vi "channel create.vi"(6 "channel classification (output data)":T1=enum."output data", 9 "data type":T2, 10 "channel name":string) -> (3 "channel":refnum<class "TBM channel.lvclass">)   [LabVIEW 2013, in "file io module configuration.lvclass"]
uses:
  file io module configuration.lvclass
  <vilib>/NI/Tag Bus/tag/Data Type.ctl
  <vilib>/NI/Tag Bus Module Framework/channel/TBM channel.lvclass
  <vilib>/NI/Tag Bus Module Framework/channel/channel classification.ctl
  <vilib>/NI/Tag Bus/tag/tag descriptor.lvclass
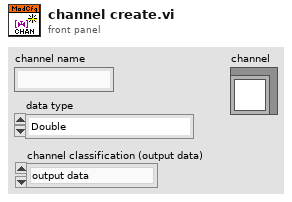
[diagram p1: front panel]
types:
  T1 = typedef "TBM channel.lvclass/channel classification.ctl" = enum16{"input data", "output data", "processing parameter", "processing result"}
  T2 = typedef "tag bus.lvlib/tag descriptor.lvclass/Data Type.ctl" = enum16{"Double", "Single", "I64", "I32", "I16", "I8", "U64", "U32", "U16", "U8", "Boolean", "String", "Array of Double", "Array of Single", "Array of I64", "Array of I32", "Array of I16", "Array of I8", "Array of U64", "Array of U32", "Array of U16", "Array of U8", "Array of Boolean", "Array of String"}
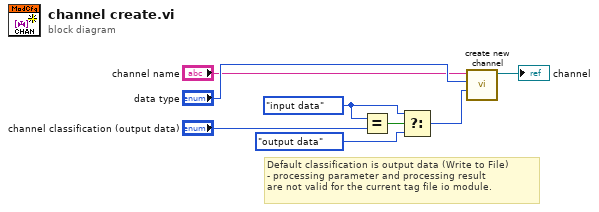
[diagram p0: block diagram]
diagram:
  w2 = channel_classification."input data" ("channel classification")
  # "Default classification is output data (Write to File) \n- processing parameter and processing result\nare not valid for the current tag file io module."
  n1 = Equal?(x=w2, y="channel classification (output data)") -> (x = y?=w5:bool)
  n2 = Select(t=w2, s=w5, f=channel_classification."output data" ("channel classification")) -> (s? t:f=w1:T1)
  n3 = call <vilib>:"create new channel.vi"("channel classification"=w1, "data type"="data type", "channel name"="channel name") -> ("channel"=→"channel":refnum<class "TBM channel.lvclass">)  [unwired: 8 in]
